vi "MM6.InitAfg.vi"(0 "i ref in":refnum<vi>, 2 "InitObjs":string[](array[string]), 3 "ms timeout (10000)":i32=10000, 4 "FreqDev":T1 {"Time" format="%.3f"; "CenterFreq" format="%.4f"; "Amp" format="%.2f"}, 5 "error in (no error)":errorcluster) -> (14 "i ref out":refnum<vi>, 16 "InitObjs out":string[](array[string]), 17 "timed out":bool, 19 "error out":errorcluster)   [LabVIEW 2014, in "MM6.lvlib"]
doc: "Initializes one AFG that may be used for anything."
uses:
  MM6.lvlib
  CSCore/CSSystem/CoreDefs/CoreDefs.call_type.ctl
  CSCore/BaseProcess/BaseProcess.descriptor string definition.ctl
  CSCore/CSSystem/CoreDefs/CoreDefs.rawDataType.ctl
  LEBITDefs/LEBITDefs.FreqDev.ctl
  CSCore/CSSystem/CoreLib/CoreLib.double 2 byte array.vi
  CSCore/BaseProcess/BaseProcess.lvlib
  LEBITLib/LEBITLib.lvlib
  CSCore/CSSystem/CoreLib/CoreLib.lvlib
  LEBITDefs/LEBITDefs.lvlib
panel:
  in  "call cluster type":T2={"Object"="", "Selector"="", "CallType"=enum."synchronous", "Async Object"="", "Async Selector"="", "Data Descriptor"="", "Data"=[], "Error #"=0, "Expire"=0}
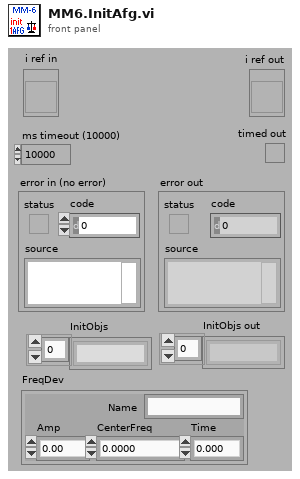
[diagram p1: front panel]
types:
  T1 = typedef "LEBITDefs.lvlib/LEBITDefs.FreqDev.ctl" = cluster{"Name":string, "Amp":dbl, "CenterFreq":dbl, "Time":dbl}
  T2 = typedef "CoreDefs.call_type.ctl" = cluster{"Object":string, "Selector":string, "CallType":enum16{"simple", "synchronous", "asynchronous"}, "Async Object":string, "Async Selector":string, "Data Descriptor":T3, "Data":T4, "Error #":i32, "Expire":u32}
  T3 = typedef "BaseProcess.lvlib/BaseProcess.descriptor string definition.ctl" = string
  T4 = typedef "CoreDefs.rawDataType.ctl" = i8[]
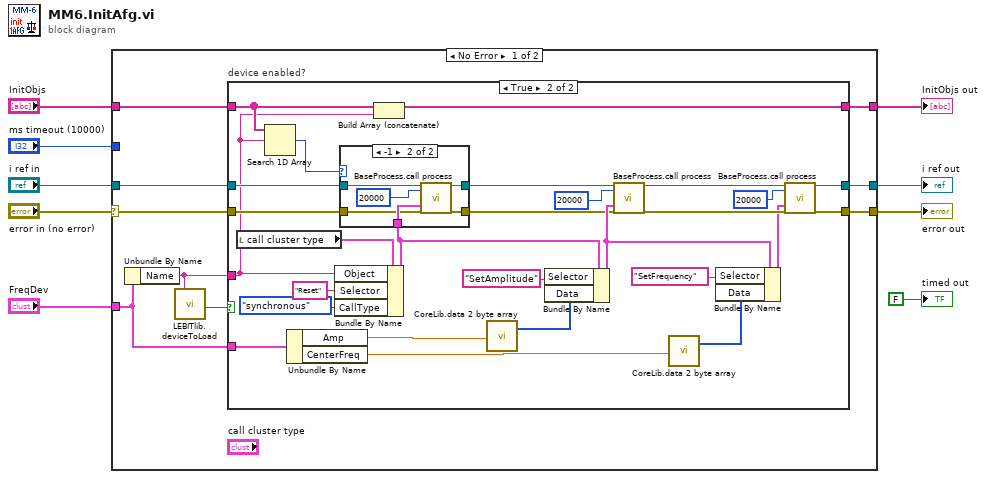
[diagram p0: block diagram]
diagram:
  n1 = case shown="No Error" "error in (no error)" {
    selector: "error in (no error)" -> [w10 w57]
    tunnel: "i ref in" -> [w11 w58]
    tunnel: [w18 w58] -> w8
    tunnel: [w17 w57] -> w7
    tunnel: "InitObjs" -> [w16 w59]
    tunnel: [w15 w59] -> w4
    tunnel: "FreqDev" -> [w12 _]
    tunnel: "ms timeout (10000)" -> [_ _]
    frame No Error {
      n2 = Unbundle By Name(w12) -> ("Name"=w13:string)
      n3 = call "LEBITlib.deviceToLoad.vi"("DeviceName"=w13) -> ("DeviceIsToLoad"=w14:bool)
      n4 = case "device enabled?" shown="True" w14 {
        tunnel: [w21 w27] -> w18
        tunnel: [w20 w26] -> w17
        tunnel: w13 -> [_ w30]
        tunnel: w12 -> [_ w36]
        tunnel: w11 -> [w21 w35]
        tunnel: w10 -> [w20 w34]
        tunnel: w16 -> [w19 w31]
        tunnel: [w19 w29] -> w15
        frame False {
        }
        frame True {
          n5 = local read "call cluster type"() -> (w43:T2)
          n6 = Search 1D Array(1D array=w31, element=w30) -> (index of element=w32:i32)  [unwired: 1 in]
          n7 = Unbundle By Name(w36) -> ("Amp"=w23:dbl, "CenterFreq"=w22:dbl)
          n8 = Bundle By Name(cluster=w43, "Object"=w30, "Selector"="Reset", "CallType"=enum16{"simple", "synchronous", "asynchronous"}."synchronous") -> (w44:T2)
          n9 = case shown="-1" w32 {
            tunnel: [w50 w55] -> w45
            tunnel: w44 -> [_ w54]
            tunnel: w35 -> [w50 w53]
            tunnel: w34 -> [w49 w52]
            tunnel: [w49 w51] -> w33
            frame 0, Default {
            }
            frame -1 {
              n10 = call "BaseProcess.call process.vi"("i ref in"=w53, "timeout (ms)"=20000, "call cluster in"=w54, "error in (no error)"=w52) -> ("i ref out"=w55:refnum<vi>, "error out"=w51:errorcluster)  [unwired: 13 in, 1 out]
            }
          }
          n11 = Build Array (concatenate)(w31, w30) -> (w29:string[])
          n12 = call-poly "CoreLib.data 2 byte array.vi"("f64"=w23) -> ("byteArray out"=w24:T4)  [unwired: 18 in]
          n13 = Bundle By Name(cluster=w44, "Selector"="SetAmplitude", "Data"=w24) -> (w40:T2)
          n14 = call "BaseProcess.call process.vi"("i ref in"=w45, "timeout (ms)"=20000, "call cluster in"=w40, "error in (no error)"=w33) -> ("i ref out"=w37:refnum<vi>, "error out"=w38:errorcluster)  [unwired: 13 in, 1 out]
          n15 = call-poly "CoreLib.data 2 byte array.vi"("f64"=w22) -> ("byteArray out"=w25:T4)  [unwired: 18 in]
          n16 = Bundle By Name(cluster=w40, "Selector"="SetFrequency", "Data"=w25) -> (w28:T2)
          n17 = call "BaseProcess.call process.vi"("i ref in"=w37, "timeout (ms)"=20000, "call cluster in"=w28, "error in (no error)"=w38) -> ("i ref out"=w27:refnum<vi>, "error out"=w26:errorcluster)  [unwired: 13 in, 1 out]
        }
      }
    }
    frame Error {
    }
  }
  "error out" <- w7
  "i ref out" <- w8
  "InitObjs out" <- w4
  "timed out" <- FALSE ("timed out")
